vi "Ideal Result.vi"(8 "Error in":errorcluster, 11 "ADC in":refnum<class "ADC.lvclass">) -> (0 "Error out":errorcluster, 3 "ADC out":refnum<class "ADC.lvclass">)   [LabVIEW 2020, in "ADC.lvclass"]
doc: "Generates Ideal values for ADC"
uses:
  ADC.lvclass
  D:/SDLC/Class/INL DNL Test/Device/Parent/Device.lvclass
  ADC.lvclass/ADC.ctl
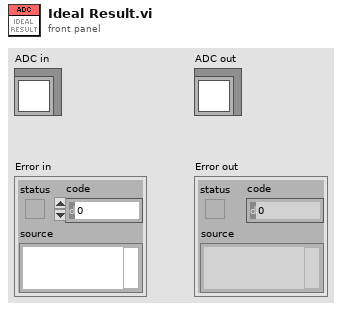
[diagram p1: front panel]
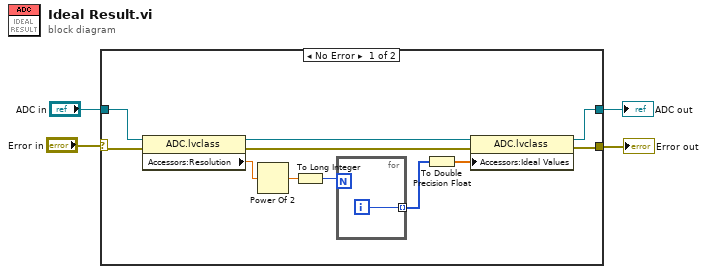
[diagram p0: block diagram]
diagram:
  n1 = case shown="No Error" "Error in" {
    selector: "Error in" -> [w14 w17]
    tunnel: "ADC in" -> [w15 w18]
    tunnel: [w8 w17] -> w2
    tunnel: [w7 w18] -> w1
    frame No Error {
      n2 = property class="ADC.lvclass"(reference=w15, error in=w14) -> (reference out=w12:refnum<class "ADC.lvclass">, error out=w11:errorcluster, "Accessors:Resolution"=w6:dbl)
      n3 = Power Of 2(x=w6) -> (2^x=w5:dbl)
      n4 = To Long Integer(number=w5) -> (32bit integer=w13:i32)
      n5 = for {
        N: w13 -> [_]
        tunnel: [w16] -> w10 mode=indexing
        i -> [w16]
      }
      n6 = To Double Precision Float(number=w10) -> (double precision float=w9:dbl[])
      n7 = property class="ADC.lvclass"(reference=w12, error in=w11, "Accessors:Ideal Values"=w9) -> (reference out=w7:refnum<class "ADC.lvclass">, error out=w8:errorcluster)
    }
    frame Error {
    }
  }
  "Error out" <- w2
  "ADC out" <- w1
